vi "Recurse Dependencies.vi"(7 "Logger":refnum<class "Logger.lvclass">, 8 "error in (no error)":errorcluster, 10 "Package":refnum<class "PackageAbstract.lvclass">, 11 "InstallAction in":refnum<class "InstallAction.lvclass">) -> (0 "error out":errorcluster, 3 "InstallAction out":refnum<class "InstallAction.lvclass">)   [LabVIEW 2020, in "GPackTools.lvlib" / "InstallAction.lvclass"]
uses:
  InstallAction.lvclass
  GPack/PackageAbstract/PackageAbstract.lvclass
  GPack/Logger/Logger.lvclass
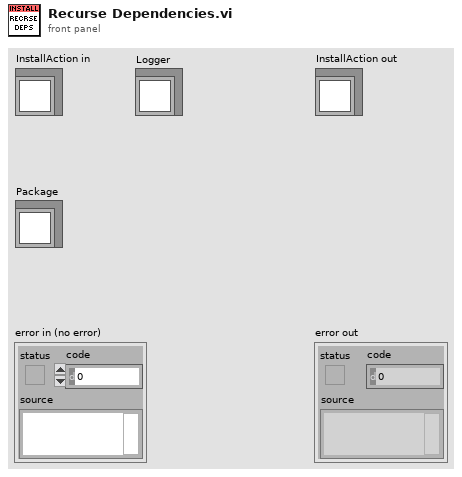
[diagram p1: front panel]
types:
  T1 = typedef "GPack.lvlib/Dependency.ctl" = cluster{"Info":T2, "Path":path}
  T2 = typedef "GPack.lvlib/Package Info.ctl" = cluster{"Name":string, "Type":string, "Host":string, "Path":string, "Branch":string, "Version":string, "License":string}
  T3 = map{string, refnum<class "PackageAbstract.lvclass">}
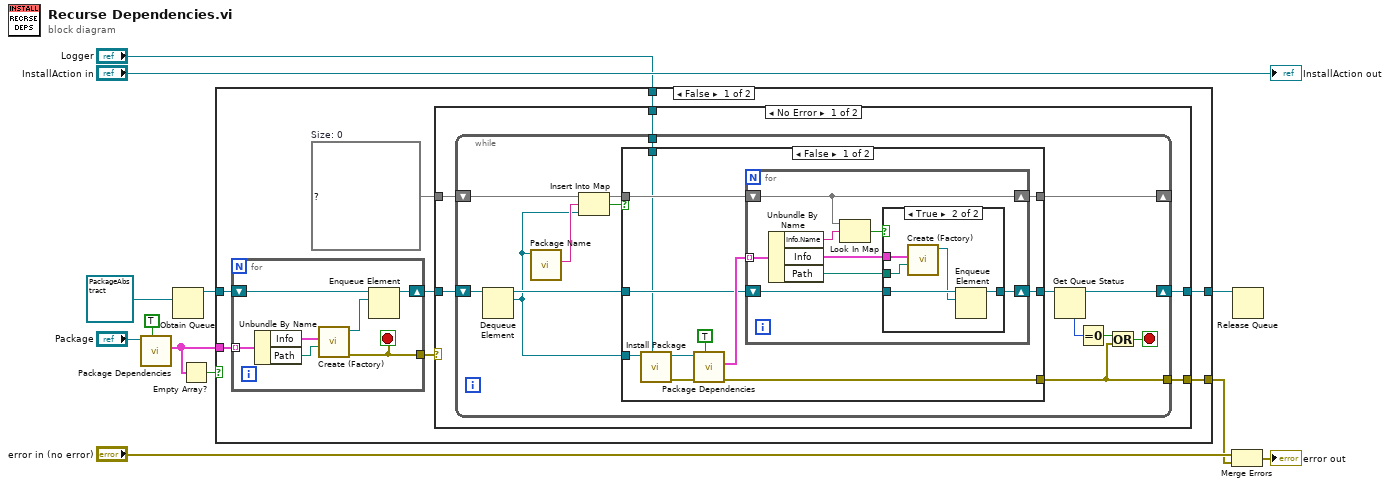
[diagram p0: block diagram]
diagram:
  n1 = call-dynamic "Package Dependencies.vi"("Absolute Path (F)"=TRUE, "PackageAbstract in"="Package") -> ("Dependencies"=w6:T1[])  [unwired: 8 in, 1 out]
  n2 = Obtain Queue(element data type=refnum<class "PackageAbstract.lvclass"> refnum ("Package")) -> (queue out=w10:refnum<queue>)  [unwired: 4 in, 2 out]
  n3 = Empty Array?(array=w6) -> (empty?=w5:bool)
  n4 = case shown="False" w5 {
    tunnel: w10 -> [w20 w77]
    tunnel: [w19 w77] -> w8
    tunnel: w6 -> [w16 _]
    tunnel: [w15 _] -> w3
    tunnel: "Logger" -> [w13 _]
    frame False {
      w17 = T3 {}  # Size: 0
      n5 = for {
        shift-right: [w26] -> w18
        shift-left: w20 -> [w27]
        tunnel: w16 -> [w25] mode=indexing
        tunnel: [w21] -> w14
        stop <- w21 stop-if-true
        n6 = Unbundle By Name(w25) -> ("Info"=w24:T2, "Path"=w23:path)
        n7 = call "Create (Factory).vi"("Folder"=w23, "Package Info"=w24) -> ("error out"=w21:errorcluster, "PackageAbstract out"=w22:refnum<class "PackageAbstract.lvclass">)  [unwired: 8 in]
        n8 = Enqueue Element(queue=w27, element=w22) -> (queue out=w26:refnum<queue>)  [unwired: 2 in, 2 out]
      }
      n9 = case shown="No Error" w14 {
        selector: w14 -> [_ w76]
        tunnel: [w32 w75] -> w19
        tunnel: w18 -> [w31 w75]
        tunnel: w17 -> [w30 _]
        tunnel: [w29 w76] -> w15
        tunnel: w13 -> [w28 _]
        frame No Error {
          n10 = while {
            tunnel: [w37] -> w29
            shift-right: [w41] -> _
            shift-left: w30 -> [w45]
            shift-right: [w40] -> w32
            shift-left: w31 -> [w47]
            tunnel: w28 -> [w33]
            stop <- w36 stop-if-true
            n11 = Dequeue Element(queue=w47) -> (queue out=w46:refnum<queue>, element=w34:refnum<class "PackageAbstract.lvclass">)  [unwired: 2 in, 2 out]
            n12 = call-dynamic "Package Name.vi"("PackageInfo in"=w34) -> ("Package Name"=w43:string)  [unwired: 9 in, 1 out]
            n13 = Insert Into Map(map in=w45, key=w43, value=w34) -> (map out=w44:T3, key already included?=w35:bool)  [unwired: 1 out]
            n14 = case shown="False" w35 {
              tunnel: w46 -> [w57 w73]
              tunnel: w44 -> [w56 w74]
              tunnel: [w55 w73] -> w42
              tunnel: [w54 w74] -> w41
              tunnel: [w53 _] -> w37
              tunnel: w34 -> [w51 _]
              tunnel: w33 -> [w48 _]
              frame False {
                n15 = call-dynamic "Install Package.vi"("Logger"=w48, "Package in"=w51) -> ("error out"=w50:errorcluster, "Package out"=w49:refnum<class "PackageAbstract.lvclass">)  [unwired: 8 in]
                n16 = call-dynamic "Package Dependencies.vi"("Absolute Path (F)"=TRUE, "error in (no error)"=w50, "PackageAbstract in"=w49) -> ("error out"=w53:errorcluster, "Dependencies"=w58:T1[])  [unwired: 7 in]
                n17 = for {
                  tunnel: w58 -> [w62] mode=indexing
                  shift-right: [w65] -> w54
                  shift-left: w56 -> [w65]
                  shift-right: [w59] -> w55
                  shift-left: w57 -> [w63]
                  n18 = Unbundle By Name(w62) -> ("Info.Name"=w66:string, "Info"=w61:T2, "Path"=w60:path)
                  n19 = Look In Map(map=w65, key=w66) -> (key not found?=w64:bool)  [unwired: 1 in, 1 out]
                  n20 = case shown="True" w64 {
                    tunnel: w63 -> [w67 w72]
                    tunnel: w61 -> [_ w71]
                    tunnel: w60 -> [_ w70]
                    tunnel: [w67 w68] -> w59
                    frame False {
                      # "Already installed"
                    }
                    frame True {
                      n21 = call "Create (Factory).vi"("Folder"=w70, "Package Info"=w71) -> ("PackageAbstract out"=w69:refnum<class "PackageAbstract.lvclass">)  [unwired: 8 in, 1 out]
                      n22 = Enqueue Element(queue=w72, element=w69) -> (queue out=w68:refnum<queue>)  [unwired: 2 in, 2 out]
                    }
                  }
                }
              }
              frame True {
              }
            }
            n23 = Get Queue Status(queue=w42) -> (queue out=w40:refnum<queue>, # elements in queue=w39:i32)  [unwired: 2 in, 6 out]
            n24 = Equal To 0?(x=w39) -> (x = 0?=w38:bool)
            n25 = Or(x=w38, y=w37) -> (x .or. y?=w36:bool)
          }
        }
        frame Error {
        }
      }
    }
    frame True {
    }
  }
  n26 = Merge Errors("error in (no error)", w3) -> (→"error out":errorcluster)
  n27 = Release Queue(queue=w8) -> ()  [unwired: 2 in, 3 out]
  "InstallAction out" <- "InstallAction in"
